vi "MultiDepth ILC Cyber Learning.vi"(0 "FPGA VI Reference In":refnum<k20>, 1 "Input RUY":T3, 2 "Change Depth?":bool, 5 "Prev Posit Cluster":T5={"Prev L1 to L4 Posit"=[-0.5319, -0.035669172703475985, -2.0566170657346783, 0.9099264705882353], "Prev Stage Posit"=[6.002553885707208, 5.996566124542428, 5.995469940427586], "Prev OCT Z Posit"=-0.0}, 7 "Learning Gains":dbl[](array[numeric])=[1.0, 1.0, 1.0, 0.0], 9 "Offset Home 2 RCM":dbl[](array[numeric])=[0.0, 0.0, 0.0, 0.0], 11 "error in":errorcluster, 12 "PID Cluster":T6={"L1 to L4 PID Cluster"={"L1 PID Gains"={"Kp"=0.005, "Kd"=0.5, "Ki"=0.0005}, "L2 PID Gains"={"Kp"=0.01, "Kd"=1.0, "Ki"=0.005}, "L3 PID Gains"={"Kp"=0.05, "Kd"=1.0, "Ki"=0.0005}, "L4 PID Gains"={"Kp"=0.1, "Kd"=0.1, "Ki"=0.0005}}, "Stage PID Cluster"={"Stage Z PID"={"Kp"=0.0005, "Kd"=0.001, "Ki"=0.0}, "Stage Y PID"={"Kp"=0.0003, "Kd"=0.01, "Ki"=0.0}, "Stage X PID"={"Kp"=0.0003, "Kd"=0.01, "Ki"=0.0}}, "OCT Z PID Gains"={"Kp"=0.0003, "Kd"=0.0001, "Ki"=0.01}}, 13 "Total Cyber Iter.":i32, 14 "Delta Ref":T2) -> (3 "Updated RUY":T3, 4 "FPGA VI Reference Out":refnum<k20>, 6 "Last Posit Cluster":T4={"Last L1 to L4 Posit"=[0.0, 0.0, 0.0, 0.0], "Last Stage Posit"=[6.0, 6.0, 6.0], "Last OCT Z Posit"=0.0}, 10 "RMS error":T1(array[cluster]), 15 "error out":errorcluster)   [LabVIEW 2016]
uses:
  <vilib>/Platform/TimedLoop/XDataNode/timing_clust.ctl
  <vilib>/Platform/TimedLoop/XDataNode/nitl_modes.ctl
  <vilib>/Platform/TimedLoop/XDataNode/wakeup.ctl
  Global Variables.vi
  <vilib>/platform/TimedLoop/XDataNode/XDataNode.xnode
  <vilib>/Platform/TimedLoop/XDataNode/XDNodeRunTimeDep.lvlib
panel:
  out "In Servo Loop":bool
  out "Loading Finished":bool
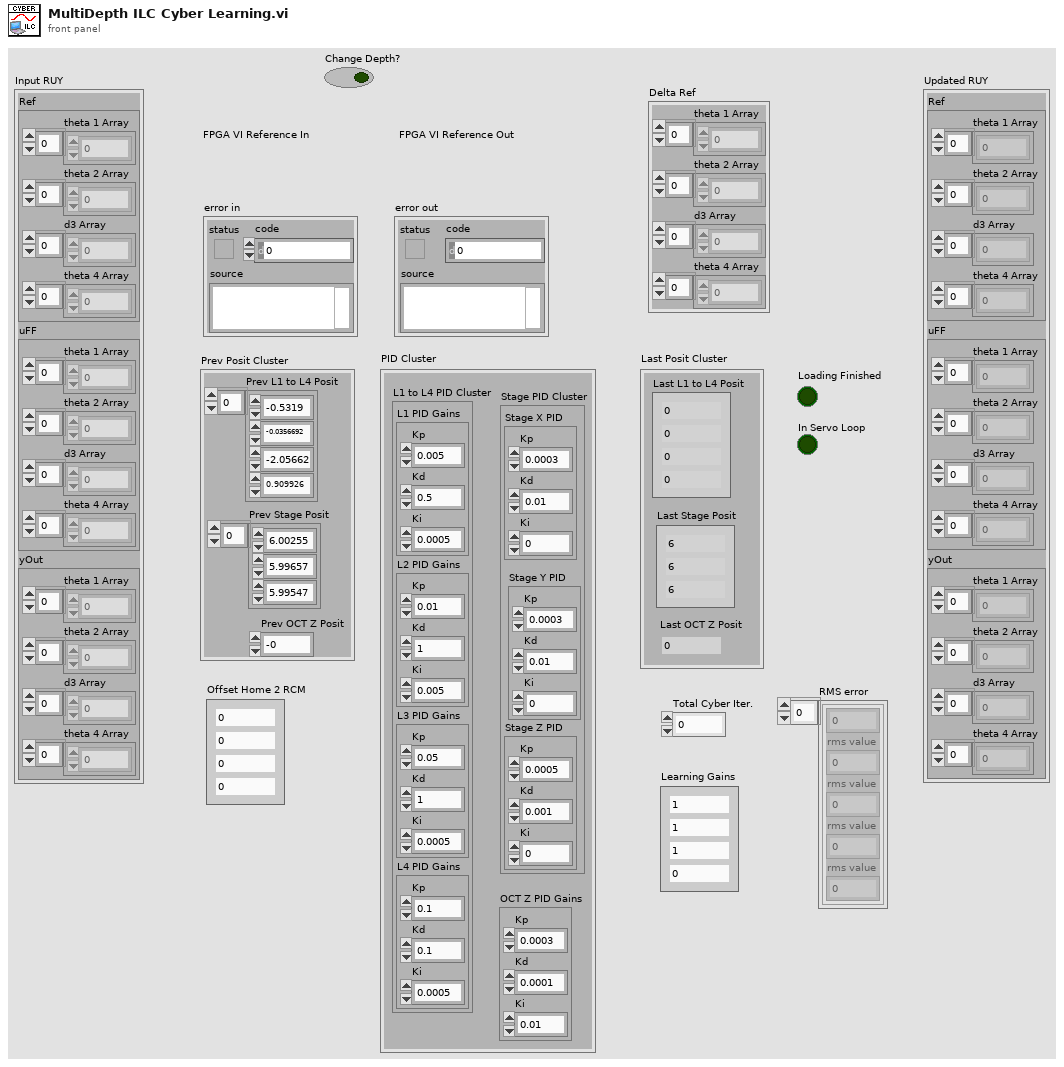
[diagram p1: front panel]
types:
  T1 = cluster{dbl, "rms value":dbl, "rms value":dbl, "rms value":dbl, "rms value":dbl}[]
  T2 = cluster{"theta 1 Array":dbl[], "theta 2 Array":dbl[], "d3 Array":dbl[], "theta 4 Array":dbl[]}
  T3 = cluster{"Ref":cluster{"theta 1 Array":dbl[], "theta 2 Array":dbl[], "d3 Array":dbl[], "theta 4 Array":dbl[]}, "uFF":cluster{"theta 1 Array":dbl[], "theta 2 Array":dbl[], "d3 Array":dbl[], "theta 4 Array":dbl[]}, "yOut":cluster{"theta 1 Array":dbl[], "theta 2 Array":dbl[], "d3 Array":dbl[], "theta 4 Array":dbl[]}}
  T4 = cluster{"Last L1 to L4 Posit":dbl[], "Last Stage Posit":dbl[], "Last OCT Z Posit":dbl}
  T5 = cluster{"Prev L1 to L4 Posit":dbl[], "Prev Stage Posit":dbl[], "Prev OCT Z Posit":dbl}
  T6 = cluster{"L1 to L4 PID Cluster":cluster{"L1 PID Gains":cluster{"Kp":dbl, "Kd":dbl, "Ki":dbl}, "L2 PID Gains":cluster{"Kp":dbl, "Kd":dbl, "Ki":dbl}, "L3 PID Gains":cluster{"Kp":dbl, "Kd":dbl, "Ki":dbl}, "L4 PID Gains":cluster{"Kp":dbl, "Kd":dbl, "Ki":dbl}}, "Stage PID Cluster":cluster{"Stage Z PID":cluster{"Kp":dbl, "Kd":dbl, "Ki":dbl}, "Stage Y PID":cluster{"Kp":dbl, "Kd":dbl, "Ki":dbl}, "Stage X PID":cluster{"Kp":dbl, "Kd":dbl, "Ki":dbl}}, "OCT Z PID Gains":cluster{"Kp":dbl, "Kd":dbl, "Ki":dbl}}
  T7 = cluster{"Stop Vacuum":bool, "Vacuum Force":i8, "Max Limit [mmHg]":dbl, "Slide in":i8, "Irrigation?":bool}
  T8 = typedef "XDNodeRunTimeDep.lvlib/timing_clust.ctl" = cluster{"Expected End [f-1]":u64, "Actual End [f-1]":u64, "Finished Late? [f-1]":bool, "Expected End [i-1]":u64, "Actual End [i-1]":u64, "Finished Late? [i-1]":bool, "Expected Start [i]":u64, "Actual Start [i]":u64, "Expected Start [f]":u64, "Actual Start [f]":u64, "Source Name":string, "Structure Name":string, "Period":i64, "Deadline":i64, "Offset":i64, "Start":i64, "Priority":i32, "Timeout":i32, "Mode":T9, "Wakeup Reason":T10, "Error":errorcluster, "Source Type":string, "Secondary Source Type":string, "Global End Time":u64, "Global Start Time":u64, "Frame Duration":u64, "Iteration Duration":u64, "Assigned CPU":i32, "I/O Scan Engine Mode":u32}
  T9 = typedef "XDNodeRunTimeDep.lvlib/nitl_modes.ctl" = enum32{"No Change", "Process missed periods, maintain original phase", "Discard missed periods, maintain original phase", "Process missed periods, ignore original phase", "Discard missed periods, ignore original phase"}
  T10 = typedef "XDNodeRunTimeDep.lvlib/wakeup.ctl" = enum32{"Normal", "Aborted", "Asynchronous wakeup", "Timing source error", "Timed loop error", "Timeout"}
  T11 = cluster{"L1 PID Gains":cluster{"Kp":dbl, "Kd":dbl, "Ki":dbl}, "L2 PID Gains":cluster{"Kp":dbl, "Kd":dbl, "Ki":dbl}, "L3 PID Gains":cluster{"Kp":dbl, "Kd":dbl, "Ki":dbl}, "L4 PID Gains":cluster{"Kp":dbl, "Kd":dbl, "Ki":dbl}}
  T12 = cluster{"Stage Z PID":cluster{"Kp":dbl, "Kd":dbl, "Ki":dbl}, "Stage Y PID":cluster{"Kp":dbl, "Kd":dbl, "Ki":dbl}, "Stage X PID":cluster{"Kp":dbl, "Kd":dbl, "Ki":dbl}}
  T13 = cluster{"Accurus button":bool[], "Accurus engaged?":bool, "Vacuum Force":i32, "Accurus Ch. A Vout":dbl, "Accurus Ch. B Vout":dbl, "Irrigation engaged?":bool}
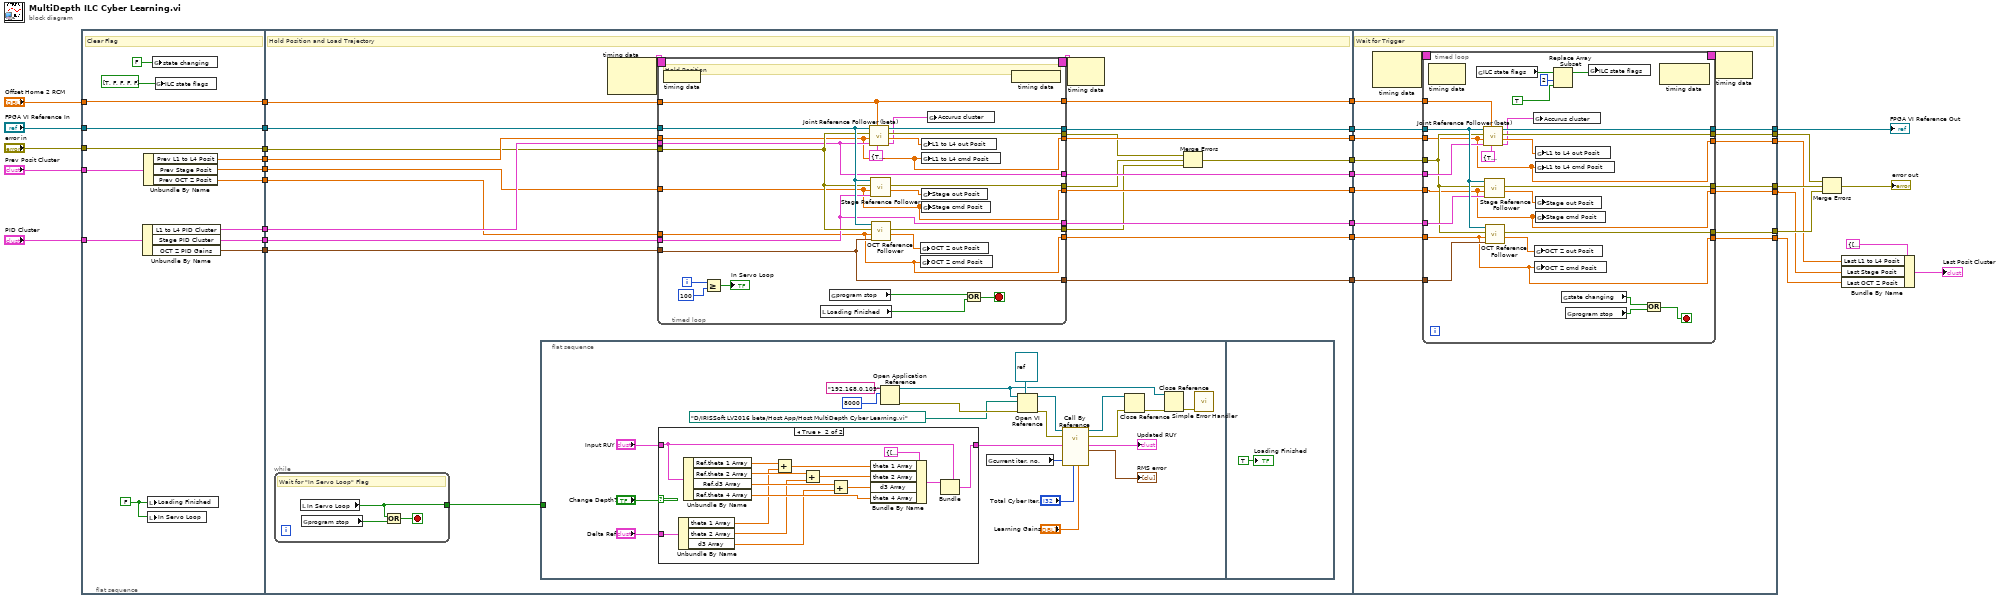
[diagram p0: block diagram]
diagram:
  n1 = flat-sequence {
    tunnel: [w46] -> w33
    tunnel: "FPGA VI Reference In" -> [w46]
    tunnel: [w45] -> w31
    tunnel: "error in" -> [w45]
    tunnel: "Prev Posit Cluster" -> [w44]
    tunnel: "PID Cluster" -> [w43]
    tunnel: [w42] -> w29
    tunnel: [w41] -> w28
    tunnel: "Offset Home 2 RCM" -> [w40]
    tunnel: [w40] -> w26
    tunnel: [w39] -> w23
    tunnel: [w38] -> w22
    tunnel: [w37] -> w21
    tunnel: [w36] -> w20
    tunnel: w33 -> [w59]
    tunnel: w31 -> [w54]
    tunnel: w29 -> [w56]
    tunnel: w28 -> [w55]
    tunnel: w26 -> [w60]
    tunnel: w23 -> [w58]
    tunnel: w22 -> [w53]
    tunnel: w21 -> [w52]
    tunnel: w20 -> [w57]
    tunnel: [w71] -> w9
    tunnel: [w70] -> w8
    tunnel: [w69] -> w7
    tunnel: [w68] -> w6
    tunnel: [w67] -> w5
    tunnel: [w66] -> w4
    tunnel: [w65] -> w3
    tunnel: [w64] -> w2
    tunnel: [w48] -> w1
    tunnel: w9 -> [w156]
    tunnel: [w155] -> w18
    tunnel: [w154] -> w17
    tunnel: [w153] -> w16
    tunnel: w8 -> [w152]
    tunnel: w7 -> [w151]
    tunnel: w6 -> [w150]
    tunnel: w5 -> [w149]
    tunnel: w4 -> [w148]
    tunnel: w3 -> [w147]
    tunnel: w2 -> [w146]
    tunnel: [w145] -> w14
    tunnel: [w144] -> w13
    tunnel: [w143] -> w12
    tunnel: [w142] -> w10
    tunnel: w1 -> [w141]
    frame #0 {
      w35 = FALSE ("Loading Finished")
      # "Clear Flag"
      n2 = Unbundle By Name(w43) -> ("L1 to L4 PID Cluster"=w41:T11, "Stage PID Cluster"=w42:T12, "OCT Z PID Gains"=w36:cluster{"Kp":dbl, "Kd":dbl, "Ki":dbl})
      n3 = Unbundle By Name(w44) -> ("Prev L1 to L4 Posit"=w39:dbl[], "Prev Stage Posit"=w38:dbl[], "Prev OCT Z Posit"=w37:dbl)
      n4 = local write "Loading Finished"(w35) -> ()
      n5 = local write "In Servo Loop"(w35) -> ()
      n6 = global write "Global Variables.vi" "state changing"(FALSE ("state changing")) -> ()
      n7 = global write "Global Variables.vi" "ILC state flags"(bool[] [TRUE, FALSE, FALSE, FALSE, FALSE]) -> ()
    }
    frame #1 {
      # "Hold Position and Load Trajectory"
      n8 = while {
        tunnel: [w73] -> w61
        stop <- w74 stop-if-true
        # "Wait for \"In Servo Loop\" Flag"
        n9 = local read "In Servo Loop"() -> (w73:bool)
        n10 = global read "Global Variables.vi" "program stop"() -> (w72:bool)
        n11 = Or(x=w73, y=w72) -> (x .or. y?=w74:bool)
      }
      n12 = flat-sequence {
        tunnel: w61 -> [_]
        frame #0 {
          n13 = case shown="True" "Change Depth?" {
            tunnel: "Input RUY" -> [w96 w98]
            tunnel: [w96 w97] -> w83
            tunnel: "Delta Ref" -> [_ w99]
            frame False {
            }
            frame True {
              n14 = Unbundle By Name(w99) -> ("theta 1 Array"=w102:dbl[], "theta 2 Array"=w103:dbl[], "d3 Array"=w104:dbl[])
              n15 = Unbundle By Name(w98) -> ("Ref.theta 1 Array"=w111:dbl[], "Ref.theta 2 Array"=w109:dbl[], "Ref.d3 Array"=w107:dbl[], "Ref.theta 4 Array"=w105:dbl[])
              n16 = Add(x=w111, y=w102) -> (x+y=w110:dbl[])
              n17 = Add(x=w109, y=w103) -> (x+y=w108:dbl[])
              n18 = Add(x=w107, y=w104) -> (x+y=w106:dbl[])
              n19 = Bundle By Name(cluster=T2 {"theta 1 Array"=[], "theta 2 Array"=[], "d3 Array"=[], "theta 4 Array"=[]} ("Ref"), "theta 1 Array"=w110, "theta 2 Array"=w108, "d3 Array"=w106, "theta 4 Array"=w105) -> (w101:T2)
              n20 = Bundle(cluster=w98, "Ref"=w101) -> (w97:T3)  [unwired: 2 in]
            }
          }
          n21 = Open Application Reference(10:u16 8000 ("port number or service name (3363)"), 11:"192.168.0.105" ("machine name (\"\":  open local reference)")) -> (0:w90:errorcluster, 3:w92:refnum<vi>)  [unwired: 2 in]
          n22 = global read "Global Variables.vi" "current iter. no."() -> (w82:u16)
          n23 = Open VI Reference(type specifier VI Refnum (for type only)=refnum<vi> refnum, application reference (local)=w92, vi path=path "D:/IRISSoft LV2016 beta/Host App/Host MultiDepth Cyber Learning.vi", error in (no error)=w90) -> (vi reference=w80:refnum<vi>, error out=w81:errorcluster)  [unwired: 2 in]
          n24 = call-by-ref "Call By Reference"(reference=w80, error in=w81, "Learning Gains"="Learning Gains", "Total Cyber Iter."="Total Cyber Iter.", "Curr Iter No"=w82, "Input RUY"=w83) -> (reference out=w77:refnum<vi>, error out=w78:errorcluster, "RMS error"=→"RMS error":T1, "Updated RUY"=→"Updated RUY":T3)  [unwired: 6 in]
          n25 = Close Reference(reference=w77, error in (no error)=w78) -> (error out=w91:errorcluster)
          n26 = Close Reference(reference=w92, error in (no error)=w91) -> (error out=w89:errorcluster)
          n27 = call <vilib>:"Simple Error Handler.vi"("error in (no error)"=w89) -> ()  [unwired: 4 in, 5 out]
        }
        frame #1 {
          "Loading Finished" <- TRUE ("Loading Finished")
        }
      }
      n28 = node-c288() -> (w63:T8)  [unwired: 2 in]
      n29 = timed-loop {
        timing: w63 -> [_]
        timing-out: [_] -> w62
        tunnel: w58 -> [w115]
        tunnel: w53 -> [w114]
        tunnel: w56 -> [w121]
        tunnel: w55 -> [w122]
        tunnel: w54 -> [w132]
        tunnel: w59 -> [w133]
        tunnel: w60 -> [w128]
        tunnel: w52 -> [w113]
        tunnel: w57 -> [w123]
        tunnel: [w115] -> w69
        tunnel: [w114] -> w68
        tunnel: [w113] -> w67
        tunnel: [w128] -> w70
        tunnel: [w127] -> w71
        tunnel: [w126] -> w51
        tunnel: [w125] -> w50
        tunnel: [w124] -> w49
        tunnel: [w123] -> w66
        tunnel: [w122] -> w65
        tunnel: [w121] -> w64
        i -> [w120]
        stop <- w136 stop-if-true
        # "Hold Position"
        n30 = node-c288 ("Output Node")() -> ()  [unwired: 1 in]
        n31 = Greater Or Equal?(x=w120, y=100) -> (x >= y?=→"In Servo Loop":bool)
        n32 = local read "Loading Finished"() -> (w135:bool)
        n33 = global read "Global Variables.vi" "program stop"() -> (w134:bool)
        n34 = call "Joint Reference Follower (beta).vi"("Accurus Ctrl Cluster"=T7 {"Stop Vacuum"=TRUE, "Vacuum Force"=0, "Max Limit [mmHg]"=600.0, "Slide in"=0, "Irrigation?"=TRUE}, "Offset Home2RCM [deg/mm]"=w128, "PID Ctrl Cluster"=w122, "Ref Array [deg/mm]"=w115, "error in"=w132, "FPGA VI Reference In"=w133) -> ("Accurus Output Cluster"=w116:T13, "Output Posit Array [deg/mm]"=w131:dbl[], "error out"=w126:errorcluster, "FPGA VI Reference Out"=w127:refnum<k20>)  [unwired: 2 in]
        n35 = call "Stage Reference Follower.vi"("Stage PID Cluster"=w121, "Stage cmd Posit [mm]"=w114, "error in"=w132, "FPGA VI Reference In"=w133) -> ("Stage out Posit [mm]"=w130:dbl[], "error out"=w125:errorcluster)  [unwired: 5 in, 1 out]
        n36 = call "OCT Reference Follower.vi"("OCT Z PID Gains"=w123, "OCT  Z cmd Posit [mm]"=w113, "error in"=w132, "FPGA VI Reference In"=w133) -> ("OCT  Z out Posit [mm]"=w129:dbl, "error out"=w124:errorcluster)  [unwired: 5 in, 1 out]
        n37 = global write "Global Variables.vi" "OCT Z out Posit"(w129) -> ()
        n38 = global write "Global Variables.vi" "OCT Z cmd Posit"(w113) -> ()
        n39 = global write "Global Variables.vi" "L1 to L4 out Posit"(w131) -> ()
        n40 = global write "Global Variables.vi" "L1 to L4 cmd Posit"(w115) -> ()
        n41 = global write "Global Variables.vi" "Stage out Posit"(w130) -> ()
        n42 = global write "Global Variables.vi" "Stage cmd Posit"(w114) -> ()
        n43 = global write "Global Variables.vi" "Accurus cluster"(w116) -> ()
        n44 = Or(x=w134, y=w135) -> (x .or. y?=w136:bool)
        n45 = node-c288() -> ()  [unwired: 1 out]
      }
      n46 = node-c288(w62) -> ()  [unwired: 1 out]
      n47 = Merge Errors(w51, w50, w49) -> (w48:errorcluster)
    }
    frame #2 {
      # "Wait for Trigger"
      n48 = node-c288() -> (w158:T8)  [unwired: 2 in]
      n49 = timed-loop {
        timing: w158 -> [_]
        timing-out: [_] -> w157
        tunnel: w156 -> [w176]
        tunnel: [w175] -> w154
        tunnel: [w174] -> w155
        tunnel: [w173] -> w153
        tunnel: w152 -> [w172]
        tunnel: w151 -> [w161]
        tunnel: w150 -> [w160]
        tunnel: w149 -> [w159]
        tunnel: w148 -> [w171]
        tunnel: w147 -> [w170]
        tunnel: w146 -> [w169]
        tunnel: [w161] -> w145
        tunnel: [w160] -> w144
        tunnel: [w159] -> w143
        tunnel: [w165] -> w142
        tunnel: w141 -> [w164]
        stop <- w183 stop-if-true
        n50 = node-c288() -> ()  [unwired: 1 in, 1 out]
        n51 = global read "Global Variables.vi" "ILC state flags"() -> (w180:bool[])
        n52 = call "Joint Reference Follower (beta).vi"("Accurus Ctrl Cluster"=T7 {"Stop Vacuum"=TRUE, "Vacuum Force"=0, "Max Limit [mmHg]"=600.0, "Slide in"=0, "Irrigation?"=TRUE}, "Offset Home2RCM [deg/mm]"=w172, "PID Ctrl Cluster"=w170, "Ref Array [deg/mm]"=w161, "error in"=w164, "FPGA VI Reference In"=w176) -> ("Accurus Output Cluster"=w162:T13, "Output Posit Array [deg/mm]"=w168:dbl[], "error out"=w175:errorcluster, "FPGA VI Reference Out"=w165:refnum<k20>)  [unwired: 2 in]
        n53 = call "Stage Reference Follower.vi"("Stage PID Cluster"=w169, "Stage cmd Posit [mm]"=w160, "error in"=w164, "FPGA VI Reference In"=w176) -> ("Stage out Posit [mm]"=w167:dbl[], "error out"=w174:errorcluster)  [unwired: 5 in, 1 out]
        n54 = call "OCT Reference Follower.vi"("OCT Z PID Gains"=w171, "OCT  Z cmd Posit [mm]"=w159, "error in"=w164, "FPGA VI Reference In"=w176) -> ("OCT  Z out Posit [mm]"=w166:dbl, "error out"=w173:errorcluster)  [unwired: 5 in, 1 out]
        n55 = global write "Global Variables.vi" "Accurus cluster"(w162) -> ()
        n56 = global write "Global Variables.vi" "OCT Z out Posit"(w166) -> ()
        n57 = global write "Global Variables.vi" "OCT Z cmd Posit"(w159) -> ()
        n58 = global write "Global Variables.vi" "L1 to L4 out Posit"(w168) -> ()
        n59 = global write "Global Variables.vi" "L1 to L4 cmd Posit"(w161) -> ()
        n60 = global write "Global Variables.vi" "Stage out Posit"(w167) -> ()
        n61 = global write "Global Variables.vi" "Stage cmd Posit"(w160) -> ()
        n62 = Replace Array Subset(array=w180, new element=TRUE ("new element/subarray"), index=2) -> (w179:bool[])
        n63 = global read "Global Variables.vi" "state changing"() -> (w182:bool)
        n64 = global read "Global Variables.vi" "program stop"() -> (w181:bool)
        n65 = global write "Global Variables.vi" "ILC state flags"(w179) -> ()
        n66 = Or(x=w182, y=w181) -> (x .or. y?=w183:bool)
        n67 = node-c288() -> ()  [unwired: 1 in, 1 out]
      }
      n68 = node-c288(w157) -> ()  [unwired: 1 out]
    }
  }
  n69 = Merge Errors(w17, w18, w16) -> (→"error out":errorcluster)
  n70 = Bundle By Name(cluster=T4 {"Last L1 to L4 Posit"=[0.0, 0.0, 0.0, 0.0], "Last Stage Posit"=[6.0, 6.0, 6.0], "Last OCT Z Posit"=0.0} ("Last Posit Cluster 2"), "Last L1 to L4 Posit"=w14, "Last Stage Posit"=w13, "Last OCT Z Posit"=w12) -> (→"Last Posit Cluster":T4)
  "FPGA VI Reference Out" <- w10
